vi "HandleObservationSync.vi"(8 "error in (no error)":errorcluster, 11 "S4GUI in":refnum<class "S4GUI.lvclass">) -> (0 "error out":errorcluster, 3 "S4GUI out":refnum<class "S4GUI.lvclass">)   [LabVIEW 2018, in "S4GUI.lvclass"] (continued)
          n762 = call "Read AcquisitionB.vi"("error in (no error)"=w1977, "S4ACS_GUI in"=w1976) -> ("error out"=w1959:errorcluster, "Acquisition.lvclass"=w1962:refnum<class "Acquisition.lvclass">, "S4ACS_GUI out"=w1963:refnum<class "S4GUI.lvclass">)  [unwired: 7 in]
          n763 = call "Read connection.vi"("error in (no error)"=w1959, "Server in"=w1962) -> ("error out"=w1958:errorcluster, "connection"=w1960:bool, "Server out"=w1961:refnum<class "Acquisition.lvclass">)  [unwired: 7 in]
          n764 = case shown="True" w1960 {
            tunnel: w1961 -> [w2040 w2056]
            tunnel: w1958 -> [w2039 w2055]
            tunnel: [w2040 w2053] -> w1957
            tunnel: [w2039 w2052] -> w1956
            tunnel: [0 ("State") w2042] -> w1926
            frame False {
            }
            frame True {
              n765 = call-dynamic "Read Channel.vi"("error in (no error)"=w2055, "Acquisition in"=w2056) -> ("error out"=w2051:errorcluster, "Channel.lvclass"=w2050:refnum<class "Channel.lvclass">, "Acquisition out"=w2054:refnum<class "Acquisition.lvclass">)  [unwired: 7 in]
              n766 = call-dynamic "Read State Machine.vi"("error in (no error)"=w2051, "Device in"=w2050) -> ("error out"=w2044:errorcluster, "State Machine.lvclass"=w2046:refnum<class "State Machine.lvclass">, "Device out"=w2048:refnum<class "Channel.lvclass">)  [unwired: 7 in]
              n767 = call-dynamic "Read State.vi"("error in (no error)"=w2044, "State Machine in"=w2046) -> ("error out"=w2043:errorcluster, "State"=w2042:i32, "State Machine out"=w2045:refnum<class "State Machine.lvclass">)  [unwired: 7 in]
              n768 = call-dynamic "Write State Machine.vi"("error in (no error)"=w2043, "State Machine.lvclass"=w2045, "Device in"=w2048) -> ("error out"=w2047:errorcluster, "Device out"=w2049:refnum<class "Channel.lvclass">)  [unwired: 7 in]
              n769 = call-dynamic "Write Channel.vi"("error in (no error)"=w2047, "Channel.lvclass"=w2049, "Acquisition in"=w2054) -> ("error out"=w2052:errorcluster, "Acquisition out"=w2053:refnum<class "Acquisition.lvclass">)  [unwired: 7 in]
            }
          }
          n770 = call "Write AcquisitionB.vi"("error in (no error)"=w1956, "Acquisition.lvclass"=w1957, "S4ACS_GUI in"=w1963) -> ("error out"=w1975:errorcluster, "S4ACS_GUI out"=w1974:refnum<class "S4GUI.lvclass">)  [unwired: 7 in]
          n771 = call-dynamic "Read AcquisitionC.vi"("error in (no error)"=w1975, "S4ACS_GUI in"=w1974) -> ("error out"=w1954:errorcluster, "Acquisition.lvclass"=w1955:refnum<class "Acquisition.lvclass">, "S4ACS_GUI out"=w1979:refnum<class "S4GUI.lvclass">)  [unwired: 7 in]
          n772 = call "Read connection.vi"("error in (no error)"=w1954, "Server in"=w1955) -> ("error out"=w1953:errorcluster, "connection"=w1951:bool, "Server out"=w1952:refnum<class "Acquisition.lvclass">)  [unwired: 7 in]
          n773 = case shown="True" w1951 {
            tunnel: w1952 -> [w2022 w2038]
            tunnel: w1953 -> [w2021 w2037]
            tunnel: [w2022 w2035] -> w1950
            tunnel: [w2021 w2034] -> w1949
            tunnel: [0 ("State") w2024] -> w1925
            frame False {
            }
            frame True {
              n774 = call-dynamic "Read Channel.vi"("error in (no error)"=w2037, "Acquisition in"=w2038) -> ("error out"=w2033:errorcluster, "Channel.lvclass"=w2032:refnum<class "Channel.lvclass">, "Acquisition out"=w2036:refnum<class "Acquisition.lvclass">)  [unwired: 7 in]
              n775 = call-dynamic "Read State Machine.vi"("error in (no error)"=w2033, "Device in"=w2032) -> ("error out"=w2026:errorcluster, "State Machine.lvclass"=w2028:refnum<class "State Machine.lvclass">, "Device out"=w2030:refnum<class "Channel.lvclass">)  [unwired: 7 in]
              n776 = call-dynamic "Read State.vi"("error in (no error)"=w2026, "State Machine in"=w2028) -> ("error out"=w2025:errorcluster, "State"=w2024:i32, "State Machine out"=w2027:refnum<class "State Machine.lvclass">)  [unwired: 7 in]
              n777 = call-dynamic "Write State Machine.vi"("error in (no error)"=w2025, "State Machine.lvclass"=w2027, "Device in"=w2030) -> ("error out"=w2029:errorcluster, "Device out"=w2031:refnum<class "Channel.lvclass">)  [unwired: 7 in]
              n778 = call-dynamic "Write Channel.vi"("error in (no error)"=w2029, "Channel.lvclass"=w2031, "Acquisition in"=w2036) -> ("error out"=w2034:errorcluster, "Acquisition out"=w2035:refnum<class "Acquisition.lvclass">)  [unwired: 7 in]
            }
          }
          n779 = call-dynamic "Write AcquisitionC.vi"("error in (no error)"=w1949, "Acquisition.lvclass"=w1950, "S4ACS_GUI in"=w1979) -> ("error out"=w1973:errorcluster, "S4ACS_GUI out"=w1972:refnum<class "S4GUI.lvclass">)  [unwired: 7 in]
          n780 = call-dynamic "Read AcquisitionD.vi"("error in (no error)"=w1973, "S4ACS_GUI in"=w1972) -> ("error out"=w1946:errorcluster, "Acquisition.lvclass"=w1948:refnum<class "Acquisition.lvclass">, "S4ACS_GUI out"=w1978:refnum<class "S4GUI.lvclass">)  [unwired: 7 in]
          n781 = call "Read connection.vi"("error in (no error)"=w1946, "Server in"=w1948) -> ("error out"=w1945:errorcluster, "connection"=w1944:bool, "Server out"=w1947:refnum<class "Acquisition.lvclass">)  [unwired: 7 in]
          n782 = case shown="True" w1944 {
            tunnel: w1947 -> [w2004 w2020]
            tunnel: w1945 -> [w2003 w2019]
            tunnel: [w2004 w2017] -> w1943
            tunnel: [w2003 w2016] -> w1942
            tunnel: [0 ("State") w2006] -> w1924
            frame False {
            }
            frame True {
              n783 = call-dynamic "Read Channel.vi"("error in (no error)"=w2019, "Acquisition in"=w2020) -> ("error out"=w2015:errorcluster, "Channel.lvclass"=w2014:refnum<class "Channel.lvclass">, "Acquisition out"=w2018:refnum<class "Acquisition.lvclass">)  [unwired: 7 in]
              n784 = call-dynamic "Read State Machine.vi"("error in (no error)"=w2015, "Device in"=w2014) -> ("error out"=w2008:errorcluster, "State Machine.lvclass"=w2010:refnum<class "State Machine.lvclass">, "Device out"=w2012:refnum<class "Channel.lvclass">)  [unwired: 7 in]
              n785 = call-dynamic "Read State.vi"("error in (no error)"=w2008, "State Machine in"=w2010) -> ("error out"=w2007:errorcluster, "State"=w2006:i32, "State Machine out"=w2009:refnum<class "State Machine.lvclass">)  [unwired: 7 in]
              n786 = call-dynamic "Write State Machine.vi"("error in (no error)"=w2007, "State Machine.lvclass"=w2009, "Device in"=w2012) -> ("error out"=w2011:errorcluster, "Device out"=w2013:refnum<class "Channel.lvclass">)  [unwired: 7 in]
              n787 = call-dynamic "Write Channel.vi"("error in (no error)"=w2011, "Channel.lvclass"=w2013, "Acquisition in"=w2018) -> ("error out"=w2016:errorcluster, "Acquisition out"=w2017:refnum<class "Acquisition.lvclass">)  [unwired: 7 in]
            }
          }
          n788 = call-dynamic "Write AcquisitionD.vi"("error in (no error)"=w1942, "Acquisition.lvclass"=w1943, "S4ACS_GUI in"=w1978) -> ("error out"=w1971:errorcluster, "S4ACS_GUI out"=w1936:refnum<class "S4GUI.lvclass">)  [unwired: 7 in]
          n789 = Equal?(x=w1928, y=w1927) -> (x = y?=w1932:bool)
          n790 = Equal?(x=w1937, y=w1927) -> (x = y?=w1941:bool)
          n791 = Equal?(x=w1928, y=w1926) -> (x = y?=w1931:bool)
          n792 = Equal?(x=w1937, y=w1926) -> (x = y?=w1940:bool)
          n793 = Equal?(x=w1928, y=w1925) -> (x = y?=w1930:bool)
          n794 = Equal?(x=w1937, y=w1925) -> (x = y?=w1939:bool)
          n795 = Equal?(x=w1928, y=w1924) -> (x = y?=w1929:bool)
          n796 = Equal?(x=w1937, y=w1924) -> (x = y?=w1938:bool)
          n797 = Compound Arithmetic op=ADD(w1927, w1926, w1925, w1924) -> (w1935:i32)
          n798 = Compound Arithmetic op=OR(w1932, w1931, w1930, w1929) -> (w1922:bool)
          n799 = Compound Arithmetic op=OR(w1941, w1940, w1939, w1938) -> (w1923:bool)
          n800 = Build Array(w1923, w1922) -> (w1921:bool[])
          n801 = Boolean Array To Number(Boolean array=w1921) -> (number=w1920:u32)
          n802 = case shown="0, Default" w1920 {
            tunnel: w1936 -> [w1986 w1994 w1998 w2002]
            tunnel: [w1985 w1993 w1997 w2001] -> w1933
            tunnel: w1935 -> [w1990 _ _ _]
            tunnel: w1934 -> [w1987 _ _ _]
            frame 0, Default {
              n803 = Equal To 0?(x=w1990) -> (x = 0?=w1989:bool)
              n804 = Select(t=u32 360, s=w1989, f=w1987) -> (s? t:f=w1984:u32)
              n805 = Bundle By Name(cluster=w1986, "Obs_state"=w1984) -> (w1985:refnum<class "S4GUI.lvclass">)
            }
            frame 1 {
              n806 = Bundle By Name(cluster=w1994, "Obs_state"=u32 1, "Error Msg"="ERROR: Some channel initialization failed. S4GUI:HandleObservationSync.vi state 272.") -> (w1993:refnum<class "S4GUI.lvclass">)
            }
            frame 2 {
              n807 = Bundle By Name(cluster=w1998, "Obs_state"=u32 1, "Error Msg"="ERROR: Some channel with invalid Exposition Time. S4GUI:HandleObservationSync.vi state 272.") -> (w1997:refnum<class "S4GUI.lvclass">)
            }
            frame 3 {
              n808 = Bundle By Name(cluster=w2002, "Obs_state"=u32 1, "Error Msg"="ERROR: Invalid configuration in the channels. S4GUI:HandleObservationSync.vi state 272.") -> (w2001:refnum<class "S4GUI.lvclass">)
            }
          }
        }
        frame 299 {
          # "Verifcando iniciação dos CICLO:"
          # "T= todos os canais ativos estão zerados."
          # "Exemplo de erro em \"Cycles_done\":\nchA; cycles_done=0; CCD_STATUS=ACTIVE;                                           Seqs_done=15;\nchA; cycles_done=0; CCD_STATUS=IDLE;                                                Seqs_done=16;   =>mudança de seq. com mesmo ciclo\nchA; cycles_done=1; CCD_STATUS=WAITING_EXPOSE_COMMAND; Seqs_done=0;\n\nchB; cycles_done=0; CCD_STATUS=ACTIVE;                                           Seqs_done=15;\nchB; cycles_done=1; CCD_STATUS=WAITING_EXPOSE_COMMAND; Seqs_done=0;     => mudança de seq com novo ciclo"
          # "T=canais receberam STOP"
          # "T= Todos os canais ativos no mesmo ciclo;\nF= Canais em ciclo diferente."
          # "Todos os CYCLES_DONE \nestão zerados?\nSe sim, vai para 327."
          # "Exemplo:\nSET #CYCLES 3\nSET #SEQ 4\ntotal de sequencias: 3 x 4 = 12\n\nseq.        CYCLES_DONE           SEQS_DONE\n1a.                     0                                 0\n2a.                     0                                 1 \n3a.                     0                                 2 \n4a.                     0                                 3 \n                          1                                 4\n5a.                     1                                 0 \n6a.                     1                                 1 \n7a.                     1                                 2 \n8a.                     1                                 3 \n                          2                                 4\n9a.                     2                                 0 \n10a.                   2                                 1 \n11a.                   2                                 2 \n12a.                   2                                 3 \n\nfim                    3                                 4"
          n809 = call-dynamic "Read AcquisitionA.vi"("error in (no error)"=w2127, "S4ACS_GUI in"=w2093) -> ("error out"=w2108:errorcluster, "Acquisition.lvclass"=w2109:refnum<class "Acquisition.lvclass">, "S4ACS_GUI out"=w2129:refnum<class "S4GUI.lvclass">)  [unwired: 7 in]
          n810 = call-dynamic "Read enabled.vi"("error in (no error)"=w2108, "Server in"=w2109) -> ("error out"=w2107:errorcluster, "enabled"=w2088:bool, "Server out"=w2106:refnum<class "Acquisition.lvclass">)  [unwired: 7 in]
          n811 = case shown="True" w2088 {
            tunnel: w2107 -> [w2219 w2235]
            tunnel: [w2220 w2233] -> w2130
            tunnel: [w2219 w2232] -> w2128
            tunnel: [u32 0 ("SequesDone") w2231] -> _
            tunnel: w2106 -> [w2220 w2230]
            tunnel: [TRUE w2229] -> w2092
            tunnel: [FALSE ("stopping") w2222] -> w2084
            frame False {
            }
            frame True {
              # "CYCLES_DONE = 0 ?"
              n812 = call-dynamic "Read Channel.vi"("error in (no error)"=w2235, "Acquisition in"=w2230) -> ("error out"=w2227:errorcluster, "Channel.lvclass"=w2228:refnum<class "Channel.lvclass">, "Acquisition out"=w2234:refnum<class "Acquisition.lvclass">)  [unwired: 7 in]
              n813 = call-dynamic "Read CyclesDone.vi"("error in (no error)"=w2227, "Channel in"=w2228) -> ("error out"=w2225:errorcluster, "CyclesDone"=w2231:u32, "Channel out"=w2226:refnum<class "Channel.lvclass">)  [unwired: 7 in]
              n814 = Equal?(x=w2231, y=u32 0) -> (x = y?=w2229:bool)
              n815 = call-dynamic "Read stopping.vi"("error in (no error)"=w2225, "Channel in"=w2226) -> ("error out"=w2224:errorcluster, "stopping"=w2222:bool, "Channel out"=w2223:refnum<class "Channel.lvclass">)  [unwired: 7 in]
              n816 = call-dynamic "Write Channel.vi"("error in (no error)"=w2224, "Channel.lvclass"=w2223, "Acquisition in"=w2234) -> ("error out"=w2232:errorcluster, "Acquisition out"=w2233:refnum<class "Acquisition.lvclass">)  [unwired: 7 in]
            }
          }
          n817 = call-dynamic "Write AcquisitionA.vi"("error in (no error)"=w2128, "Acquisition.lvclass"=w2130, "S4ACS_GUI in"=w2129) -> ("error out"=w2125:errorcluster, "S4ACS_GUI out"=w2124:refnum<class "S4GUI.lvclass">)  [unwired: 7 in]
          n818 = call "Read AcquisitionB.vi"("error in (no error)"=w2125, "S4ACS_GUI in"=w2124) -> ("error out"=w2102:errorcluster, "Acquisition.lvclass"=w2105:refnum<class "Acquisition.lvclass">, "S4ACS_GUI out"=w2126:refnum<class "S4GUI.lvclass">)  [unwired: 7 in]
          n819 = call-dynamic "Read enabled.vi"("error in (no error)"=w2102, "Server in"=w2105) -> ("error out"=w2103:errorcluster, "enabled"=w2087:bool, "Server out"=w2104:refnum<class "Acquisition.lvclass">)  [unwired: 7 in]
          n820 = case shown="True" w2087 {
            tunnel: w2103 -> [w2199 w2215]
            tunnel: w2104 -> [w2200 w2214]
            tunnel: [u32 0 ("SequesDone") w2209] -> _
            tunnel: [w2199 w2213] -> w2123
            tunnel: [w2200 w2212] -> w2122
            tunnel: [TRUE w2208] -> w2091
            tunnel: [FALSE ("stopping") w2202] -> w2083
            frame False {
            }
            frame True {
              n821 = call-dynamic "Read Channel.vi"("error in (no error)"=w2215, "Acquisition in"=w2214) -> ("error out"=w2206:errorcluster, "Channel.lvclass"=w2207:refnum<class "Channel.lvclass">, "Acquisition out"=w2210:refnum<class "Acquisition.lvclass">)  [unwired: 7 in]
              n822 = call-dynamic "Read CyclesDone.vi"("error in (no error)"=w2206, "Channel in"=w2207) -> ("error out"=w2204:errorcluster, "CyclesDone"=w2209:u32, "Channel out"=w2211:refnum<class "Channel.lvclass">)  [unwired: 7 in]
              n823 = Equal?(x=w2209, y=u32 0) -> (x = y?=w2208:bool)
              n824 = call-dynamic "Read stopping.vi"("error in (no error)"=w2204, "Channel in"=w2211) -> ("error out"=w2203:errorcluster, "stopping"=w2202:bool, "Channel out"=w2205:refnum<class "Channel.lvclass">)  [unwired: 7 in]
              n825 = call-dynamic "Write Channel.vi"("error in (no error)"=w2203, "Channel.lvclass"=w2205, "Acquisition in"=w2210) -> ("error out"=w2213:errorcluster, "Acquisition out"=w2212:refnum<class "Acquisition.lvclass">)  [unwired: 7 in]
            }
          }
          n826 = call "Write AcquisitionB.vi"("error in (no error)"=w2123, "Acquisition.lvclass"=w2122, "S4ACS_GUI in"=w2126) -> ("error out"=w2115:errorcluster, "S4ACS_GUI out"=w2114:refnum<class "S4GUI.lvclass">)  [unwired: 7 in]
          n827 = call-dynamic "Read AcquisitionC.vi"("error in (no error)"=w2115, "S4ACS_GUI in"=w2114) -> ("error out"=w2099:errorcluster, "Acquisition.lvclass"=w2101:refnum<class "Acquisition.lvclass">, "S4ACS_GUI out"=w2117:refnum<class "S4GUI.lvclass">)  [unwired: 7 in]
          n828 = call-dynamic "Read enabled.vi"("error in (no error)"=w2099, "Server in"=w2101) -> ("error out"=w2098:errorcluster, "enabled"=w2086:bool, "Server out"=w2100:refnum<class "Acquisition.lvclass">)  [unwired: 7 in]
          n829 = case shown="True" w2086 {
            tunnel: [w2179 w2195] -> w2118
            tunnel: [w2180 w2194] -> w2116
            tunnel: w2098 -> [w2179 w2191]
            tunnel: w2100 -> [w2180 w2192]
            tunnel: [u32 0 ("SequesDone") w2190] -> _
            tunnel: [TRUE w2189] -> w2090
            tunnel: [FALSE ("stopping") w2182] -> w2082
            frame False {
            }
            frame True {
              n830 = call-dynamic "Read Channel.vi"("error in (no error)"=w2191, "Acquisition in"=w2192) -> ("error out"=w2186:errorcluster, "Channel.lvclass"=w2187:refnum<class "Channel.lvclass">, "Acquisition out"=w2193:refnum<class "Acquisition.lvclass">)  [unwired: 7 in]
              n831 = call-dynamic "Read CyclesDone.vi"("error in (no error)"=w2186, "Channel in"=w2187) -> ("error out"=w2184:errorcluster, "CyclesDone"=w2190:u32, "Channel out"=w2188:refnum<class "Channel.lvclass">)  [unwired: 7 in]
              n832 = Equal?(x=w2190, y=u32 0) -> (x = y?=w2189:bool)
              n833 = call-dynamic "Read stopping.vi"("error in (no error)"=w2184, "Channel in"=w2188) -> ("error out"=w2183:errorcluster, "stopping"=w2182:bool, "Channel out"=w2185:refnum<class "Channel.lvclass">)  [unwired: 7 in]
              n834 = call-dynamic "Write Channel.vi"("error in (no error)"=w2183, "Channel.lvclass"=w2185, "Acquisition in"=w2193) -> ("error out"=w2195:errorcluster, "Acquisition out"=w2194:refnum<class "Acquisition.lvclass">)  [unwired: 7 in]
            }
          }
          n835 = call-dynamic "Write AcquisitionC.vi"("error in (no error)"=w2118, "Acquisition.lvclass"=w2116, "S4ACS_GUI in"=w2117) -> ("error out"=w2112:errorcluster, "S4ACS_GUI out"=w2113:refnum<class "S4GUI.lvclass">)  [unwired: 7 in]
          n836 = call-dynamic "Read AcquisitionD.vi"("error in (no error)"=w2112, "S4ACS_GUI in"=w2113) -> ("error out"=w2095:errorcluster, "Acquisition.lvclass"=w2097:refnum<class "Acquisition.lvclass">, "S4ACS_GUI out"=w2119:refnum<class "S4GUI.lvclass">)  [unwired: 7 in]
          n837 = call-dynamic "Read enabled.vi"("error in (no error)"=w2095, "Server in"=w2097) -> ("error out"=w2094:errorcluster, "enabled"=w2085:bool, "Server out"=w2096:refnum<class "Acquisition.lvclass">)  [unwired: 7 in]
          n838 = case shown="True" w2085 {
            tunnel: [w2160 w2175] -> w2121
            tunnel: [w2159 w2174] -> w2120
            tunnel: w2096 -> [w2160 w2173]
            tunnel: w2094 -> [w2159 w2172]
            tunnel: [u32 0 ("SequesDone") w2170] -> _
            tunnel: [TRUE w2169] -> w2089
            tunnel: [FALSE ("stopping") w2162] -> w2081
            frame False {
            }
            frame True {
              n839 = call-dynamic "Read Channel.vi"("error in (no error)"=w2172, "Acquisition in"=w2173) -> ("error out"=w2166:errorcluster, "Channel.lvclass"=w2167:refnum<class "Channel.lvclass">, "Acquisition out"=w2171:refnum<class "Acquisition.lvclass">)  [unwired: 7 in]
              n840 = call-dynamic "Read CyclesDone.vi"("error in (no error)"=w2166, "Channel in"=w2167) -> ("error out"=w2164:errorcluster, "CyclesDone"=w2170:u32, "Channel out"=w2168:refnum<class "Channel.lvclass">)  [unwired: 7 in]
              n841 = Equal?(x=w2170, y=u32 0) -> (x = y?=w2169:bool)
              n842 = call-dynamic "Read stopping.vi"("error in (no error)"=w2164, "Channel in"=w2168) -> ("error out"=w2163:errorcluster, "stopping"=w2162:bool, "Channel out"=w2165:refnum<class "Channel.lvclass">)  [unwired: 7 in]
              n843 = call-dynamic "Write Channel.vi"("error in (no error)"=w2163, "Channel.lvclass"=w2165, "Acquisition in"=w2171) -> ("error out"=w2174:errorcluster, "Acquisition out"=w2175:refnum<class "Acquisition.lvclass">)  [unwired: 7 in]
            }
          }
          n844 = Compound Arithmetic op=AND(w2092, w2091, w2090, w2089) -> (w2078:bool)
          n845 = Compound Arithmetic op=OR(w2084, w2083, w2082, w2081) -> (w2080:bool)
          n846 = call-dynamic "Write AcquisitionD.vi"("error in (no error)"=w2120, "Acquisition.lvclass"=w2121, "S4ACS_GUI in"=w2119) -> ("error out"=w2110:errorcluster, "S4ACS_GUI out"=w2111:refnum<class "S4GUI.lvclass">)  [unwired: 7 in]
          n847 = case shown="True" w2078 {
            tunnel: w2111 -> [w2141 w2152]
            tunnel: [w2140 w2151] -> w2079
            tunnel: w2080 -> [_ w2150]
            tunnel: w2077 -> [_ w2147]
            frame False {
              # "Esperando todos os canais habilitados mudarem de cyclesDone.\nE verificando a maior duracao de cubo entre os canais."
              n848 = local read "time307"() -> (w2139:u32)
              n849 = Tick Count (ms)() -> (millisecond timer value=w2138:u32)
              n850 = Subtract(x=w2138, y=w2139) -> (x-y=w2134:u32)
              n851 = call-dynamic "GetGreatestCube.vi"("S4GUI in"=w2141) -> ("S4GUI out"=w2136:refnum<class "S4GUI.lvclass">, "greatest (ms)"=w2132:dbl)  [unwired: 8 in, 1 out]
              n852 = To Double Precision Float(number=w2134) -> (double precision float=w2137:dbl)
              n853 = Add(x=1000.0 ("y"), y=w2132) -> (x+y=w2131:dbl)
              n854 = Less?(x=w2131, y=w2137) -> (x < y?=w2135:bool)
              n855 = case shown="False" w2135 {
                tunnel: w2136 -> [w2142 w2146]
                tunnel: [w2142 w2145] -> w2140
                frame False {
                }
                frame True {
                  n856 = Bundle By Name(cluster=w2146, "Obs_state"=u32 1, "Error Msg"="ERROR: Cycles_Done reseting timeout. - HandleObservationSync.vi state 299.") -> (w2145:refnum<class "S4GUI.lvclass">)
                }
              }
            }
            frame True {
              # "STOP?"
              n857 = case shown="False" w2150 {
                tunnel: [w2153 u32 0] -> w2149
                tunnel: w2147 -> [w2154 _]
                frame False {
                  n858 = Increment(x=w2154) -> (x+1=w2153:u32)
                }
                frame True {
                }
              }
              n859 = Bundle By Name(cluster=w2152, "Obs_state"=w2149, "cyclesDone"=u32 0) -> (w2151:refnum<class "S4GUI.lvclass">)
            }
          }
        }
        frame 300 {
          # "Verifica se é modo fotometria ou polarimetria:\nTrue = polarimetria (esatdo 301)\nFalse = fotometria (estado 321)"
          n860 = flat-sequence {
            tunnel: w2240 -> [w2253]
            tunnel: [w2253] -> w2239
            frame #0 {
              n861 = local read "time3"() -> (w2255:u32)
              n862 = local read "time4"() -> (w2252:u32)
              n863 = Tick Count (ms)() -> (millisecond timer value=w2251:u32)
              n864 = Subtract(x=w2252, y=w2255) -> (x-y=→"delay 3-4":u32)
              n865 = local write "time1"(w2251) -> ()
            }
          }
          n866 = call "Read Instrument.lvclass.vi"("error in (no error)"=w2239, "S4ACS_GUI in"=w2250) -> ("error out"=w2245:errorcluster, "Instrument.lvclass"=w2246:refnum<class "Instrument.lvclass">, "S4ACS_GUI out"=w2244:refnum<class "S4GUI.lvclass">)  [unwired: 7 in]
          n867 = call-dynamic "Read mode.vi"("error in (no error)"=w2245, "Instrument in"=w2246) -> ("error out"=w2241:errorcluster, "mode"=w2243:bool)  [unwired: 7 in, 1 out]
          n868 = Select(t=u32 301, s=w2243, f=u32 321 ("t")) -> (s? t:f=w2248:u32)
          n869 = Bundle By Name(cluster=w2244, "Obs_state"=w2248, "cyclesDone"=u32 0, "sequesDone"=u32 0, "seqAtual"=u32 0) -> (w2249:refnum<class "S4GUI.lvclass">)
        }
        frame 301 {
          # "Configurando para ACS esperar comando EXPOSE"
          n870 = call-dynamic "Read AcquisitionA.vi"("error in (no error)"=w2318, "S4ACS_GUI in"=w2319) -> ("error out"=w2273:errorcluster, "Acquisition.lvclass"=w2274:refnum<class "Acquisition.lvclass">, "S4ACS_GUI out"=w2321:refnum<class "S4GUI.lvclass">)  [unwired: 7 in]
          n871 = call-dynamic "Read enabled.vi"("error in (no error)"=w2273, "Server in"=w2274) -> ("error out"=w2272:errorcluster, "enabled"=w2259:bool, "Server out"=w2275:refnum<class "Acquisition.lvclass">)  [unwired: 7 in]
          n872 = call "Read connection.vi"("error in (no error)"=w2272, "Server in"=w2275) -> ("error out"=w2298:errorcluster, "connection"=w2282:bool, "Server out"=w2299:refnum<class "Acquisition.lvclass">)  [unwired: 7 in]
          n873 = And(x=w2282, y=w2259) -> (x .and. y?=w2283:bool)
          n874 = case shown="True" w2283 {
            tunnel: w2299 -> [w2436 w2455]
            tunnel: w2298 -> [w2435 w2454]
            tunnel: [w2436 w2452] -> w2322
            tunnel: [w2435 w2451] -> w2320
            tunnel: [w2432 u32 0 ("New_State")] -> w2288
            tunnel: w2259 -> [w2431 _]
            frame False {
              n875 = Select(t=u32 1, s=w2431, f=u32 0) -> (s? t:f=w2432:u32)
            }
            frame True {
              n876 = call-dynamic "Read Channel.vi"("error in (no error)"=w2454, "Acquisition in"=w2455) -> ("error out"=w2438:errorcluster, "Channel.lvclass"=w2441:refnum<class "Channel.lvclass">, "Acquisition out"=w2453:refnum<class "Acquisition.lvclass">)  [unwired: 7 in]
              n877 = call-dynamic "Write wait_expose.vi"("error in (no error)"=w2438, "wait_expose"=TRUE, "Channel in"=w2441) -> ("error out"=w2437:errorcluster, "Channel out"=w2440:refnum<class "Channel.lvclass">)  [unwired: 7 in]
              n878 = call-dynamic "Read State Machine.vi"("error in (no error)"=w2437, "Device in"=w2440) -> ("error out"=w2448:errorcluster, "State Machine.lvclass"=w2450:refnum<class "State Machine.lvclass">, "Device out"=w2446:refnum<class "Channel.lvclass">)  [unwired: 7 in]
              n879 = call "Next State.vi"("error in (no error)"=w2448, "New_State"=40, "State Machine in"=w2450) -> ("error out"=w2443:errorcluster, "State Machine out"=w2444:refnum<class "State Machine.lvclass">)  [unwired: 7 in]
              n880 = call-dynamic "Write State Machine.vi"("error in (no error)"=w2443, "State Machine.lvclass"=w2444, "Device in"=w2446) -> ("error out"=w2445:errorcluster, "Device out"=w2447:refnum<class "Channel.lvclass">)  [unwired: 7 in]
              n881 = call-dynamic "Write Channel.vi"("error in (no error)"=w2445, "Channel.lvclass"=w2447, "Acquisition in"=w2453) -> ("error out"=w2451:errorcluster, "Acquisition out"=w2452:refnum<class "Acquisition.lvclass">)  [unwired: 7 in]
            }
          }
          n882 = call-dynamic "Write AcquisitionA.vi"("error in (no error)"=w2320, "Acquisition.lvclass"=w2322, "S4ACS_GUI in"=w2321) -> ("error out"=w2315:errorcluster, "S4ACS_GUI out"=w2316:refnum<class "S4GUI.lvclass">)  [unwired: 7 in]
          n883 = call "Read AcquisitionB.vi"("error in (no error)"=w2315, "S4ACS_GUI in"=w2316) -> ("error out"=w2269:errorcluster, "Acquisition.lvclass"=w2271:refnum<class "Acquisition.lvclass">, "S4ACS_GUI out"=w2313:refnum<class "S4GUI.lvclass">)  [unwired: 7 in]
          n884 = call-dynamic "Read enabled.vi"("error in (no error)"=w2269, "Server in"=w2271) -> ("error out"=w2268:errorcluster, "enabled"=w2258:bool, "Server out"=w2270:refnum<class "Acquisition.lvclass">)  [unwired: 7 in]
          n885 = call "Read connection.vi"("error in (no error)"=w2268, "Server in"=w2270) -> ("error out"=w2296:errorcluster, "connection"=w2280:bool, "Server out"=w2297:refnum<class "Acquisition.lvclass">)  [unwired: 7 in]
          n886 = And(x=w2280, y=w2258) -> (x .and. y?=w2281:bool)
          n887 = case shown="False" w2281 {
            tunnel: w2297 -> [w2411 w2430]
            tunnel: w2296 -> [w2410 w2429]
            tunnel: [w2411 w2427] -> w2314
            tunnel: [w2410 w2426] -> w2312
            tunnel: [w2407 u32 0 ("New_State")] -> w2287
            tunnel: w2258 -> [w2406 _]
            frame False {
              n888 = Select(t=u32 2, s=w2406, f=u32 0) -> (s? t:f=w2407:u32)
            }
            frame True {
              n889 = call-dynamic "Read Channel.vi"("error in (no error)"=w2429, "Acquisition in"=w2430) -> ("error out"=w2413:errorcluster, "Channel.lvclass"=w2415:refnum<class "Channel.lvclass">, "Acquisition out"=w2428:refnum<class "Acquisition.lvclass">)  [unwired: 7 in]
              n890 = call-dynamic "Write wait_expose.vi"("error in (no error)"=w2413, "wait_expose"=TRUE, "Channel in"=w2415) -> ("error out"=w2412:errorcluster, "Channel out"=w2414:refnum<class "Channel.lvclass">)  [unwired: 7 in]
              n891 = call-dynamic "Read State Machine.vi"("error in (no error)"=w2412, "Device in"=w2414) -> ("error out"=w2423:errorcluster, "State Machine.lvclass"=w2425:refnum<class "State Machine.lvclass">, "Device out"=w2421:refnum<class "Channel.lvclass">)  [unwired: 7 in]
              n892 = call "Next State.vi"("error in (no error)"=w2423, "New_State"=40, "State Machine in"=w2425) -> ("error out"=w2418:errorcluster, "State Machine out"=w2419:refnum<class "State Machine.lvclass">)  [unwired: 7 in]
              n893 = call-dynamic "Write State Machine.vi"("error in (no error)"=w2418, "State Machine.lvclass"=w2419, "Device in"=w2421) -> ("error out"=w2420:errorcluster, "Device out"=w2422:refnum<class "Channel.lvclass">)  [unwired: 7 in]
              n894 = call-dynamic "Write Channel.vi"("error in (no error)"=w2420, "Channel.lvclass"=w2422, "Acquisition in"=w2428) -> ("error out"=w2426:errorcluster, "Acquisition out"=w2427:refnum<class "Acquisition.lvclass">)  [unwired: 7 in]
            }
          }
          n895 = call "Write AcquisitionB.vi"("error in (no error)"=w2312, "Acquisition.lvclass"=w2314, "S4ACS_GUI in"=w2313) -> ("error out"=w2308:errorcluster, "S4ACS_GUI out"=w2307:refnum<class "S4GUI.lvclass">)  [unwired: 7 in]
          n896 = call-dynamic "Read AcquisitionC.vi"("error in (no error)"=w2308, "S4ACS_GUI in"=w2307) -> ("error out"=w2265:errorcluster, "Acquisition.lvclass"=w2267:refnum<class "Acquisition.lvclass">, "S4ACS_GUI out"=w2310:refnum<class "S4GUI.lvclass">)  [unwired: 7 in]
          n897 = call-dynamic "Read enabled.vi"("error in (no error)"=w2265, "Server in"=w2267) -> ("error out"=w2264:errorcluster, "enabled"=w2257:bool, "Server out"=w2266:refnum<class "Acquisition.lvclass">)  [unwired: 7 in]
          n898 = call "Read connection.vi"("error in (no error)"=w2264, "Server in"=w2266) -> ("error out"=w2294:errorcluster, "connection"=w2277:bool, "Server out"=w2295:refnum<class "Acquisition.lvclass">)  [unwired: 7 in]
          n899 = And(x=w2277, y=w2257) -> (x .and. y?=w2279:bool)
          n900 = case shown="True" w2279 {
            tunnel: [w2385 w2399] -> w2311
            tunnel: [w2386 w2398] -> w2309
            tunnel: w2295 -> [w2386 w2396]
            tunnel: w2294 -> [w2385 w2395]
            tunnel: [w2382 u32 0 ("New_State")] -> w2286
            tunnel: w2257 -> [w2381 _]
            frame False {
              n901 = Select(t=u32 4, s=w2381, f=u32 0) -> (s? t:f=w2382:u32)
            }
            frame True {
              n902 = call-dynamic "Read Channel.vi"("error in (no error)"=w2395, "Acquisition in"=w2396) -> ("error out"=w2388:errorcluster, "Channel.lvclass"=w2390:refnum<class "Channel.lvclass">, "Acquisition out"=w2397:refnum<class "Acquisition.lvclass">)  [unwired: 7 in]
              n903 = call-dynamic "Write wait_expose.vi"("error in (no error)"=w2388, "wait_expose"=TRUE, "Channel in"=w2390) -> ("error out"=w2387:errorcluster, "Channel out"=w2389:refnum<class "Channel.lvclass">)  [unwired: 7 in]
              n904 = call-dynamic "Read State Machine.vi"("error in (no error)"=w2387, "Device in"=w2389) -> ("error out"=w2402:errorcluster, "State Machine.lvclass"=w2400:refnum<class "State Machine.lvclass">, "Device out"=w2404:refnum<class "Channel.lvclass">)  [unwired: 7 in]
              n905 = call "Next State.vi"("error in (no error)"=w2402, "New_State"=40, "State Machine in"=w2400) -> ("error out"=w2394:errorcluster, "State Machine out"=w2393:refnum<class "State Machine.lvclass">)  [unwired: 7 in]
              n906 = call-dynamic "Write State Machine.vi"("error in (no error)"=w2394, "State Machine.lvclass"=w2393, "Device in"=w2404) -> ("error out"=w2405:errorcluster, "Device out"=w2403:refnum<class "Channel.lvclass">)  [unwired: 7 in]
              n907 = call-dynamic "Write Channel.vi"("error in (no error)"=w2405, "Channel.lvclass"=w2403, "Acquisition in"=w2397) -> ("error out"=w2399:errorcluster, "Acquisition out"=w2398:refnum<class "Acquisition.lvclass">)  [unwired: 7 in]
            }
          }
          n908 = call-dynamic "Write AcquisitionC.vi"("error in (no error)"=w2311, "Acquisition.lvclass"=w2309, "S4ACS_GUI in"=w2310) -> ("error out"=w2305:errorcluster, "S4ACS_GUI out"=w2304:refnum<class "S4GUI.lvclass">)  [unwired: 7 in]
          n909 = call-dynamic "Read AcquisitionD.vi"("error in (no error)"=w2305, "S4ACS_GUI in"=w2304) -> ("error out"=w2261:errorcluster, "Acquisition.lvclass"=w2263:refnum<class "Acquisition.lvclass">, "S4ACS_GUI out"=w2303:refnum<class "S4GUI.lvclass">)  [unwired: 7 in]
          n910 = call-dynamic "Read enabled.vi"("error in (no error)"=w2261, "Server in"=w2263) -> ("error out"=w2260:errorcluster, "enabled"=w2256:bool, "Server out"=w2262:refnum<class "Acquisition.lvclass">)  [unwired: 7 in]
          n911 = call "Read connection.vi"("error in (no error)"=w2260, "Server in"=w2262) -> ("error out"=w2292:errorcluster, "connection"=w2276:bool, "Server out"=w2293:refnum<class "Acquisition.lvclass">)  [unwired: 7 in]
          n912 = And(x=w2276, y=w2256) -> (x .and. y?=w2278:bool)
          n913 = case shown="True" w2278 {
            tunnel: w2292 -> [w2360 w2380]
            tunnel: [w2360 w2379] -> w2306
            tunnel: w2293 -> [w2361 w2372]
            tunnel: [w2361 w2370] -> w2302
            tunnel: [w2357 u32 0 ("New_State")] -> w2285
            tunnel: w2256 -> [w2356 _]
            frame False {
              n914 = Select(t=u32 8, s=w2356, f=u32 0) -> (s? t:f=w2357:u32)
            }
            frame True {
              n915 = call-dynamic "Read Channel.vi"("error in (no error)"=w2380, "Acquisition in"=w2372) -> ("error out"=w2362:errorcluster, "Channel.lvclass"=w2365:refnum<class "Channel.lvclass">, "Acquisition out"=w2371:refnum<class "Acquisition.lvclass">)  [unwired: 7 in]
              n916 = call-dynamic "Write wait_expose.vi"("error in (no error)"=w2362, "wait_expose"=TRUE, "Channel in"=w2365) -> ("error out"=w2363:errorcluster, "Channel out"=w2364:refnum<class "Channel.lvclass">)  [unwired: 7 in]
              n917 = call-dynamic "Read State Machine.vi"("error in (no error)"=w2363, "Device in"=w2364) -> ("error out"=w2376:errorcluster, "State Machine.lvclass"=w2378:refnum<class "State Machine.lvclass">, "Device out"=w2374:refnum<class "Channel.lvclass">)  [unwired: 7 in]
              n918 = call "Next State.vi"("error in (no error)"=w2376, "New_State"=40, "State Machine in"=w2378) -> ("error out"=w2368:errorcluster, "State Machine out"=w2369:refnum<class "State Machine.lvclass">)  [unwired: 7 in]
              n919 = call-dynamic "Write State Machine.vi"("error in (no error)"=w2368, "State Machine.lvclass"=w2369, "Device in"=w2374) -> ("error out"=w2373:errorcluster, "Device out"=w2375:refnum<class "Channel.lvclass">)  [unwired: 7 in]
              n920 = call-dynamic "Write Channel.vi"("error in (no error)"=w2373, "Channel.lvclass"=w2375, "Acquisition in"=w2371) -> ("error out"=w2379:errorcluster, "Acquisition out"=w2370:refnum<class "Acquisition.lvclass">)  [unwired: 7 in]
            }
          }
          n921 = call-dynamic "Write AcquisitionD.vi"("error in (no error)"=w2306, "Acquisition.lvclass"=w2302, "S4ACS_GUI in"=w2303) -> ("error out"=w2301:errorcluster, "S4ACS_GUI out"=w2300:refnum<class "S4GUI.lvclass">)  [unwired: 7 in]
          n922 = Compound Arithmetic op=ADD(w2288, w2287, w2286, w2285) -> (w2289:u32)
          n923 = case shown="0, Default" w2289 {
            tunnel: w2284 -> [w2325 _ _ _ _ _ _ _ _ _ _ _ _ _ _ _]
            tunnel: [w2324 u32 1 ("Obs_state") u32 1 ("Obs_state") u32 1 ("Obs_state") u32 1 ("Obs_state") u32 1 ("Obs_state") u32 1 ("Obs_state") u32 1 ("Obs_state") u32 1 ("Obs_state") u32 1 ("Obs_state") u32 1 ("Obs_state") u32 1 ("Obs_state") u32 1 ("Obs_state") u32 1 ("Obs_state") u32 1 ("Obs_state") u32 1 ("Obs_state")] -> w2290
            tunnel: ["" ("Error Msg") "ERROR: Lost channel 1 connection... - HandleObservationSync.vi state 301" ("Error Msg") "ERROR: Lost channel 2 connection...- HandleObservationSync.vi state 301" ("Error Msg") "ERROR: Lost channels 1 and 2 connection...- HandleObservationSync.vi state 301" ("Error Msg") "ERROR: Lost channel 3 connection...- HandleObservationSync.vi state 301" ("Error Msg") "ERROR: Lost channels 1 and  3 connection...- HandleObservationSync.vi state 301" ("Error Msg") "ERROR:  Lost channels 2 and  3 connection...- HandleObservationSync.vi state 301" ("Error Msg") "ERROR:  Lost channels 1, 2 and  3 connection...- HandleObservationSync.vi state 301" ("Error Msg") "ERROR: Lost channel 4 connection...- HandleObservationSync.vi state 301" ("Error Msg") "ERROR:  Lost channels 1 and 4 connection...- HandleObservationSync.vi state 301" ("Error Msg") "ERROR:  Lost channels 2 and 4 connection...- HandleObservationSync.vi state 301" ("Error Msg") "ERROR: Lost channels 1, 2 and 4 connection...- HandleObservationSync.vi state 301" ("Error Msg") "ERROR: Lost channels 3 and 4 connection...- HandleObservationSync.vi state 301" ("Error Msg") "ERROR: Lost channels 1, 3 and 4 connection...- HandleObservationSync.vi state 301" ("Error Msg") "ERROR: Lost channels 2, 3 and 4 connection...- HandleObservationSync.vi state 301" ("Error Msg") "ERROR: Lost channels 1, 2, 3 and 4 connection...- HandleObservationSync.vi state 301" ("Error Msg")] -> w2291
            frame 0, Default {
              n924 = Increment(x=w2325) -> (x+1=w2324:u32)
            }
            frame 1 {
            }
            frame 2 {
            }
            frame 3 {
            }
            frame 4 {
            }
            frame 5 {
            }
            frame 6 {
            }
            frame 7 {
            }
            frame 8 {
            }
            frame 9 {
            }
            frame 10 {
            }
            frame 11 {
            }
            frame 12 {
            }
            frame 13 {
            }
            frame 14 {
            }
            frame 15 {
            }
          }
          n925 = Bundle By Name(cluster=w2300, "Obs_state"=w2290, "Error Msg"=w2291) -> (w2317:refnum<class "S4GUI.lvclass">)
        }
        frame 302 {
          # "Espera terminar o envio de WAIT EXPOSE COMMAND para todos os ACS."
          n926 = call-dynamic "VerifyAcqIdle.vi"("error in (no error)"=w2457, "S4GUI in"=w2456) -> ("error out"=w2462:errorcluster, "idle"=w2461:bool, "S4GUI out"=w2463:refnum<class "S4GUI.lvclass">)  [unwired: 6 in, 1 out]
          n927 = Increment(x=w2459) -> (x+1=w2458:u32)
          n928 = Select(t=w2458, s=w2461, f=w2459) -> (s? t:f=w2460:u32)
          n929 = Bundle By Name(cluster=w2463, "Obs_state"=w2460) -> (w2464:refnum<class "S4GUI.lvclass">)
        }
        frame 303 {
          n930 = flat-sequence {
            tunnel: w2470 -> [w2509]
            tunnel: [w2509] -> w2469
            frame #0 {
              n931 = Tick Count (ms)() -> (millisecond timer value=→"time1":u32)
            }
          }
          n932 = call "Read Instrument.lvclass.vi"("error in (no error)"=w2469, "S4ACS_GUI in"=w2505) -> ("error out"=w2507:errorcluster, "Instrument.lvclass"=w2508:refnum<class "Instrument.lvclass">, "S4ACS_GUI out"=w2466:refnum<class "S4GUI.lvclass">)  [unwired: 7 in]
          n933 = call "Read WPROT.vi"("error in (no error)"=w2507, "Instrument in"=w2508) -> ("error out"=w2498:errorcluster, "Opt_Selector.lvclass"=w2499:refnum<class "Opt_Selector.lvclass">, "Instrument out"=w2506:refnum<class "Instrument.lvclass">)  [unwired: 7 in]
          n934 = call-dynamic "getTargetPos.vi"("error in (no error)"=w2498, "Opt_Selector in"=w2499) -> ("error out"=w2497:errorcluster, "Target Pos"=w2477:u16, "Opt_Selector out"=w2496:refnum<class "Opt_Selector.lvclass">)  [unwired: 7 in]
          n935 = Unbundle By Name(w2466) -> ("seqAtual"=w2468:u32)
          n936 = Build Array(-1.0 ("element"), 0.0 ("element"), 22.5 ("element"), 45.0 ("element"), 67.5 ("element"), 90.0 ("element"), 112.5 ("element"), 135.0 ("element"), 157.5 ("element"), 180.0 ("element"), 202.5 ("element"), 225.0 ("element"), 247.5 ("element"), 270.0 ("element"), 292.5 ("element"), 315.0 ("element"), 337.5 ("element")) -> (w2489:dbl[])
          n937 = Index Array(array=w2489, index=w2477) -> (element=w2476:dbl)
          n938 = case shown="1..16" w2477 {
            selector: w2477 -> [_ w2543]
            tunnel: w2506 -> [w2519 w2531]
            tunnel: [w2519 w2531] -> w2472
            tunnel: [w2516 w2530] -> w2471
            tunnel: w2502 -> [_ w2545]
            tunnel: [u32 314 w2544] -> w2501
            tunnel: w2497 -> [w2517 w2539]
            tunnel: w2496 -> [w2518 w2538]
            tunnel: w2476 -> [_ w2533]
            tunnel: [w2514 w2532] -> w2473
            tunnel: [u32 0 w2521] -> w2467
            tunnel: w2468 -> [_ w2522]
            frame 0, Default {
              # "Terminou uma sequência.\nRecupera as posições em SEQ e desvia para 314 para verificar se há mais ciclos."
              # "Recupera a sequencia anterior para o caso \nde repetição da sequencia (sem precisar clicar \nnas posicoes desejadas novamente)."
              n939 = call-dynamic "Read sequencia_ant.vi"("error in (no error)"=w2517, "Opt_Selector in"=w2518) -> ("error out"=w2513:errorcluster, "sequencia_ant"=w2512:u16, "Opt_Selector out"=w2515:refnum<class "Opt_Selector.lvclass">)  [unwired: 7 in]
              n940 = call-dynamic "Write sequencia.vi"("error in (no error)"=w2513, "sequencia"=w2512, "Opt_Selector in"=w2515) -> ("error out"=w2516:errorcluster, "Opt_Selector out"=w2514:refnum<class "Opt_Selector.lvclass">)  [unwired: 7 in]
            }
            frame 1..16 {
              # "Inicia o Ticks com\nvalor do relogio atual"
              # "Espera até 40 x 0.25s (= 10s) para\nmecanismo entrar em READY"
              n941 = Number To Decimal String(number=w2543) -> (decimal integer string=w2542:string)  [unwired: 1 in]
              n942 = Concatenate Strings("WP" ("string"), w2542) -> (w2540:string)
              n943 = call "Write target name.vi"("error in (no error)"=w2539, "target name"=w2540, "Optics in"=w2538) -> ("error out"=w2536:errorcluster, "Optics out"=w2537:refnum<class "Opt_Selector.lvclass">)  [unwired: 7 in]
              n944 = call "Write target.vi"("error in (no error)"=w2536, "target"=w2533, "Optics in"=w2537) -> ("error out"=w2535:errorcluster, "Optics out"=w2534:refnum<class "Opt_Selector.lvclass">)  [unwired: 7 in]
              n945 = call-dynamic "Read State Machine.vi"("error in (no error)"=w2535, "Device in"=w2534) -> ("error out"=w2547:errorcluster, "State Machine.lvclass"=w2549:refnum<class "State Machine.lvclass">, "Device out"=w2546:refnum<class "Opt_Selector.lvclass">)  [unwired: 7 in]
              n946 = Increment(x=w2545) -> (x+1=w2544:u32)
              n947 = call "Next State.vi"("error in (no error)"=w2547, "New_State"=1, "State Machine in"=w2549) -> ("error out"=w2528:errorcluster, "State Machine out"=w2529:refnum<class "State Machine.lvclass">)  [unwired: 7 in]
              n948 = Increment(x=w2522) -> (x+1=w2521:u32)
              n949 = call-dynamic "Write Timer.vi"("error in (no error)"=w2528, "Timer"=u32 40, "State Machine in"=w2529) -> ("error out"=w2525:errorcluster, "State Machine out"=w2526:refnum<class "State Machine.lvclass">)  [unwired: 7 in]
              n950 = call-dynamic "Init Ticks2.vi"("error in (no error)"=w2525, "State Machine in"=w2526) -> ("error out"=w2524:errorcluster, "State Machine out"=w2523:refnum<class "State Machine.lvclass">)  [unwired: 8 in]
              n951 = call-dynamic "Write State Machine.vi"("error in (no error)"=w2524, "State Machine.lvclass"=w2523, "Device in"=w2546) -> ("error out"=w2530:errorcluster, "Device out"=w2532:refnum<class "Opt_Selector.lvclass">)  [unwired: 7 in]
            }
          }
          n952 = Bundle By Name(cluster=w2466, "seqAtual"=w2467) -> (w2465:refnum<class "S4GUI.lvclass">)
          n953 = call "Write WPROT.vi"("error in (no error)"=w2471, "Opt_Selector.lvclass"=w2473, "Instrument in"=w2472) -> ("error out"=w2475:errorcluster, "Instrument out"=w2474:refnum<class "Instrument.lvclass">)  [unwired: 7 in]
          n954 = call "Write Instrument.lvclass.vi"("error in (no error)"=w2475, "Instrument.lvclass"=w2474, "S4ACS_GUI in"=w2465) -> ("error out"=w2504:errorcluster, "S4ACS_GUI out"=w2503:refnum<class "S4GUI.lvclass">)  [unwired: 7 in]
          n955 = Bundle By Name(cluster=w2503, "Obs_state"=w2501) -> (w2500:refnum<class "S4GUI.lvclass">)
        }
        frame 304 {
          # "Para inserir Pausa antes do\nEXPOSE, ir para 305."
          # "Espera terminar o movimento da lamina para disparar a aquisição\ndos canais ativos.\n\nOV 20230424: Não precisa mais atualizar o valor de WPPOS com o\ncomando WRITE_HEADER porque o ACS já recebeu a sequência de\nposições da lâmina."
          n956 = flat-sequence {
            tunnel: w2577 -> [w2604]
            tunnel: [w2604] -> w2576
            frame #0 {
              n957 = Tick Count (ms)() -> (millisecond timer value=w2603:u32)
              "time 2" <- w2603
              n958 = local read "time1"() -> (w2602:u32)
              n959 = Subtract(x=w2603, y=w2602) -> (x-y=→"delay wp":u32)
            }
          }
          n960 = call "Read Instrument.lvclass.vi"("error in (no error)"=w2576, "S4ACS_GUI in"=w2584) -> ("error out"=w2589:errorcluster, "Instrument.lvclass"=w2590:refnum<class "Instrument.lvclass">, "S4ACS_GUI out"=w2586:refnum<class "S4GUI.lvclass">)  [unwired: 7 in]
          n961 = call "Read WPROT.vi"("error in (no error)"=w2589, "Instrument in"=w2590) -> ("error out"=w2583:errorcluster, "Opt_Selector.lvclass"=w2582:refnum<class "Opt_Selector.lvclass">, "Instrument out"=w2588:refnum<class "Instrument.lvclass">)  [unwired: 7 in]
          n962 = call-dynamic "Read State Machine.vi"("error in (no error)"=w2583, "Device in"=w2582) -> ("error out"=w2561:errorcluster, "State Machine.lvclass"=w2564:refnum<class "State Machine.lvclass">, "Device out"=w2580:refnum<class "Opt_Selector.lvclass">)  [unwired: 7 in]
          n963 = call-dynamic "Verif Clock 2.vi"("error in (no error)"=w2561, "period (ms)"=u32 20000 ("period"), "State Machine in"=w2564) -> ("error out"=w2560:errorcluster, "time elapsed"=→"time elapsed":u32, "State Machine out"=w2563:refnum<class "State Machine.lvclass">)  [unwired: 6 in]
          n964 = call-dynamic "Read Timeout 2.vi"("error in (no error)"=w2560, "State Machine in"=w2563) -> ("error out"=w2559:errorcluster, "Timeout 2"=w2565:bool, "State Machine out"=w2562:refnum<class "State Machine.lvclass">)  [unwired: 7 in]
          n965 = call-dynamic "Read State.vi"("error in (no error)"=w2559, "State Machine in"=w2562) -> ("error out"=w2574:errorcluster, "State"=w2578:i32, "State Machine out"=w2575:refnum<class "State Machine.lvclass">)  [unwired: 7 in]
          n966 = Equal To 0?(x=w2578) -> (x = 0?=w2552:bool)
          n967 = call-dynamic "Write State Machine.vi"("error in (no error)"=w2574, "State Machine.lvclass"=w2575, "Device in"=w2580) -> ("error out"=w2579:errorcluster, "Device out"=w2581:refnum<class "Opt_Selector.lvclass">)  [unwired: 7 in]
          n968 = call "Write WPROT.vi"("error in (no error)"=w2579, "Opt_Selector.lvclass"=w2581, "Instrument in"=w2588) -> ("error out"=w2585:errorcluster, "Instrument out"=w2587:refnum<class "Instrument.lvclass">)  [unwired: 7 in]
          n969 = call "Write Instrument.lvclass.vi"("error in (no error)"=w2585, "Instrument.lvclass"=w2587, "S4ACS_GUI in"=w2586) -> ("error out"=w2567:errorcluster, "S4ACS_GUI out"=w2558:refnum<class "S4GUI.lvclass">)  [unwired: 7 in]
          n970 = case shown="True" w2565 {
            tunnel: w2553 -> [w2593 _]
            tunnel: [w2593 u32 1 ("Obs_state")] -> w2554
            tunnel: w2558 -> [w2592 w2598]
            tunnel: [w2592 w2597] -> w2557
            tunnel: [w2591 FALSE] -> w2551
            tunnel: w2552 -> [w2591 _]
            frame False {
            }
            frame True {
              n971 = Bundle By Name(cluster=w2598, "Error Msg"="ERROR: moving waveplate timeout  (S4GUI:HandleObservationSync.vi - state 302)") -> (w2597:refnum<class "S4GUI.lvclass">)
            }
          }
          n972 = Unbundle By Name(w2558) -> ("cyclesDone"=w2571:u32, "seqAtual"=w2570:u32)
          n973 = Decrement(x=w2570) -> (x-1=w2555:u32)
          n974 = Add(x=w2571, y=w2555) -> (x+y=w2569:u32)
          n975 = Equal To 0?(x=w2569) -> (x = 0?=w2572:bool)
          n976 = Increment(x=w2553) -> ()  [unwired: 1 out]
          n977 = case shown="True" w2572 {
            tunnel: [u32 308 ("t") u32 308 ("t")] -> w2550
            frame False {
              (unwired) u32 310 ("t")
              # "Não é 1a seq:\nvai direto para\nenvio do trigger"
            }
            frame True {
              # "1a sequencia:\nenvia EXPOSE"
            }
          }
          n978 = Select(t=w2550, s=w2551, f=w2554) -> (s? t:f=w2573:u32)
          n979 = Bundle By Name(cluster=w2557, "Obs_state"=w2573) -> (w2568:refnum<class "S4GUI.lvclass">)
        }
        frame 305 {
          # "Pausa de 200ms entre o posicionamento da \nlâmina e o envio de EXPOSE para o ACS."
          n980 = flat-sequence {
            tunnel: w2616 -> [w2623]
            tunnel: [w2623] -> w2608
            frame #0 {
              n981 = Tick Count (ms)() -> (millisecond timer value=w2621:u32)
              n982 = local read "time1"() -> (w2622:u32)
              n983 = Subtract(x=w2621, y=w2622) -> (x-y=w2620:u32)
              n984 = local write "delay wp"(w2620) -> ()
            }
          }
          n985 = Tick Count (ms)() -> (millisecond timer value=w2605:u32)
          n986 = local read "time 2"() -> (w2611:u32)
          n987 = Subtract(x=w2605, y=w2611) -> (x-y=w2613:u32)
          n988 = To Double Precision Float(number=w2613) -> (double precision float=w2614:dbl)
          n989 = Less?(x=200.0 ("y"), y=w2614) -> (x < y?=w2610:bool)
          n990 = case shown="True" w2610 {
            tunnel: [w2617 u32 308 ("t")] -> w2607
            tunnel: w2606 -> [w2617 _]
            tunnel: w2605 -> [_ w2618]
            frame False {
            }
            frame True {
              # "1a sequencia:\nenvia EXPOSE"
              n991 = local write "time 2"(w2618) -> ()
            }
          }
          n992 = Bundle By Name(cluster=w2609, "Obs_state"=w2607) -> (w2615:refnum<class "S4GUI.lvclass">)
        }
        frame 308 {
          n993 = call-dynamic "Read AcquisitionA.vi"("error in (no error)"=w2686, "S4ACS_GUI in"=w2687) -> ("error out"=w2641:errorcluster, "Acquisition.lvclass"=w2642:refnum<class "Acquisition.lvclass">, "S4ACS_GUI out"=w2689:refnum<class "S4GUI.lvclass">)  [unwired: 7 in]
          n994 = call-dynamic "Read enabled.vi"("error in (no error)"=w2641, "Server in"=w2642) -> ("error out"=w2640:errorcluster, "enabled"=w2627:bool, "Server out"=w2643:refnum<class "Acquisition.lvclass">)  [unwired: 7 in]
          n995 = call "Read connection.vi"("error in (no error)"=w2640, "Server in"=w2643) -> ("error out"=w2666:errorcluster, "connection"=w2650:bool, "Server out"=w2667:refnum<class "Acquisition.lvclass">)  [unwired: 7 in]
          n996 = And(x=w2650, y=w2627) -> (x .and. y?=w2651:bool)
          n997 = case shown="True" w2651 {
            tunnel: w2667 -> [w2796 w2812]
            tunnel: w2666 -> [w2795 w2811]
            tunnel: [w2796 w2809] -> w2690
            tunnel: [w2795 w2808] -> w2688
            tunnel: [w2792 u32 0 ("New_State")] -> w2656
            tunnel: w2627 -> [w2791 _]
            frame False {
              n998 = Select(t=u32 1, s=w2791, f=u32 0) -> (s? t:f=w2792:u32)
            }
            frame True {
              n999 = call-dynamic "Read Channel.vi"("error in (no error)"=w2811, "Acquisition in"=w2812) -> ("error out"=w2804:errorcluster, "Channel.lvclass"=w2803:refnum<class "Channel.lvclass">, "Acquisition out"=w2810:refnum<class "Acquisition.lvclass">)  [unwired: 7 in]
              n1000 = call-dynamic "Read State Machine.vi"("error in (no error)"=w2804, "Device in"=w2803) -> ("error out"=w2805:errorcluster, "State Machine.lvclass"=w2807:refnum<class "State Machine.lvclass">, "Device out"=w2801:refnum<class "Channel.lvclass">)  [unwired: 7 in]
              n1001 = call "Next State.vi"("error in (no error)"=w2805, "New_State"=50, "State Machine in"=w2807) -> ("error out"=w2798:errorcluster, "State Machine out"=w2799:refnum<class "State Machine.lvclass">)  [unwired: 7 in]
              n1002 = call-dynamic "Write State Machine.vi"("error in (no error)"=w2798, "State Machine.lvclass"=w2799, "Device in"=w2801) -> ("error out"=w2800:errorcluster, "Device out"=w2802:refnum<class "Channel.lvclass">)  [unwired: 7 in]
              n1003 = call-dynamic "Write Channel.vi"("error in (no error)"=w2800, "Channel.lvclass"=w2802, "Acquisition in"=w2810) -> ("error out"=w2808:errorcluster, "Acquisition out"=w2809:refnum<class "Acquisition.lvclass">)  [unwired: 7 in]
            }
          }
          n1004 = call-dynamic "Write AcquisitionA.vi"("error in (no error)"=w2688, "Acquisition.lvclass"=w2690, "S4ACS_GUI in"=w2689) -> ("error out"=w2683:errorcluster, "S4ACS_GUI out"=w2684:refnum<class "S4GUI.lvclass">)  [unwired: 7 in]
          n1005 = call "Read AcquisitionB.vi"("error in (no error)"=w2683, "S4ACS_GUI in"=w2684) -> ("error out"=w2637:errorcluster, "Acquisition.lvclass"=w2639:refnum<class "Acquisition.lvclass">, "S4ACS_GUI out"=w2681:refnum<class "S4GUI.lvclass">)  [unwired: 7 in]
          n1006 = call-dynamic "Read enabled.vi"("error in (no error)"=w2637, "Server in"=w2639) -> ("error out"=w2636:errorcluster, "enabled"=w2626:bool, "Server out"=w2638:refnum<class "Acquisition.lvclass">)  [unwired: 7 in]
          n1007 = call "Read connection.vi"("error in (no error)"=w2636, "Server in"=w2638) -> ("error out"=w2664:errorcluster, "connection"=w2648:bool, "Server out"=w2665:refnum<class "Acquisition.lvclass">)  [unwired: 7 in]
          n1008 = And(x=w2648, y=w2626) -> (x .and. y?=w2649:bool)
          n1009 = case shown="True" w2649 {
            tunnel: w2665 -> [w2774 w2790]
            tunnel: w2664 -> [w2773 w2789]
            tunnel: [w2774 w2787] -> w2682
            tunnel: [w2773 w2786] -> w2680
            tunnel: [w2770 u32 0 ("New_State")] -> w2655
            tunnel: w2626 -> [w2769 _]
            frame False {
              n1010 = Select(t=u32 2, s=w2769, f=u32 0) -> (s? t:f=w2770:u32)
            }
            frame True {
              n1011 = call-dynamic "Read Channel.vi"("error in (no error)"=w2789, "Acquisition in"=w2790) -> ("error out"=w2782:errorcluster, "Channel.lvclass"=w2781:refnum<class "Channel.lvclass">, "Acquisition out"=w2788:refnum<class "Acquisition.lvclass">)  [unwired: 7 in]
              n1012 = call-dynamic "Read State Machine.vi"("error in (no error)"=w2782, "Device in"=w2781) -> ("error out"=w2783:errorcluster, "State Machine.lvclass"=w2785:refnum<class "State Machine.lvclass">, "Device out"=w2779:refnum<class "Channel.lvclass">)  [unwired: 7 in]
              n1013 = call "Next State.vi"("error in (no error)"=w2783, "New_State"=50, "State Machine in"=w2785) -> ("error out"=w2776:errorcluster, "State Machine out"=w2777:refnum<class "State Machine.lvclass">)  [unwired: 7 in]
              n1014 = call-dynamic "Write State Machine.vi"("error in (no error)"=w2776, "State Machine.lvclass"=w2777, "Device in"=w2779) -> ("error out"=w2778:errorcluster, "Device out"=w2780:refnum<class "Channel.lvclass">)  [unwired: 7 in]
              n1015 = call-dynamic "Write Channel.vi"("error in (no error)"=w2778, "Channel.lvclass"=w2780, "Acquisition in"=w2788) -> ("error out"=w2786:errorcluster, "Acquisition out"=w2787:refnum<class "Acquisition.lvclass">)  [unwired: 7 in]
            }
          }
          n1016 = call "Write AcquisitionB.vi"("error in (no error)"=w2680, "Acquisition.lvclass"=w2682, "S4ACS_GUI in"=w2681) -> ("error out"=w2676:errorcluster, "S4ACS_GUI out"=w2675:refnum<class "S4GUI.lvclass">)  [unwired: 7 in]
          n1017 = call-dynamic "Read AcquisitionC.vi"("error in (no error)"=w2676, "S4ACS_GUI in"=w2675) -> ("error out"=w2633:errorcluster, "Acquisition.lvclass"=w2635:refnum<class "Acquisition.lvclass">, "S4ACS_GUI out"=w2678:refnum<class "S4GUI.lvclass">)  [unwired: 7 in]
          n1018 = call-dynamic "Read enabled.vi"("error in (no error)"=w2633, "Server in"=w2635) -> ("error out"=w2632:errorcluster, "enabled"=w2625:bool, "Server out"=w2634:refnum<class "Acquisition.lvclass">)  [unwired: 7 in]
          n1019 = call "Read connection.vi"("error in (no error)"=w2632, "Server in"=w2634) -> ("error out"=w2662:errorcluster, "connection"=w2645:bool, "Server out"=w2663:refnum<class "Acquisition.lvclass">)  [unwired: 7 in]
          n1020 = And(x=w2645, y=w2625) -> (x .and. y?=w2647:bool)
          n1021 = case shown="True" w2647 {
            tunnel: [w2751 w2760] -> w2679
            tunnel: [w2752 w2759] -> w2677
            tunnel: w2663 -> [w2752 w2757]
            tunnel: w2662 -> [w2751 w2756]
            tunnel: [w2748 u32 0 ("New_State")] -> w2654
            tunnel: w2625 -> [w2747 _]
            frame False {
              n1022 = Select(t=u32 4, s=w2747, f=u32 0) -> (s? t:f=w2748:u32)
            }
            frame True {
              n1023 = call-dynamic "Read Channel.vi"("error in (no error)"=w2756, "Acquisition in"=w2757) -> ("error out"=w2764:errorcluster, "Channel.lvclass"=w2765:refnum<class "Channel.lvclass">, "Acquisition out"=w2758:refnum<class "Acquisition.lvclass">)  [unwired: 7 in]
